vi "JME Test Solutions Visa Device Simulator.vi"() -> ()   [LabVIEW 2020]
doc: "This VI will wait for a TCP Connection and then respond to TCP Reqests based on the responses list"
panel:
  in  "Enable?":bool
  in  "Responses Config":string[][](array[string])
  in  "Load Button":bool
  in  "Responses File":path
  in  "stop":bool
  in  "port":u16=50000
  in  "Stop Button":bool
  # "JME Test Solutions VISA Device Simulator"
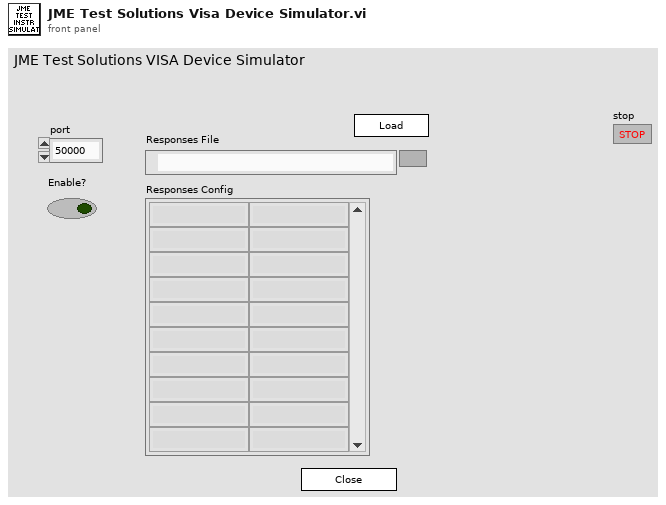
[diagram p1: front panel]
types:
  T1 = enum16{"Standard", "Buffered", "CRLF", "Immediate"}
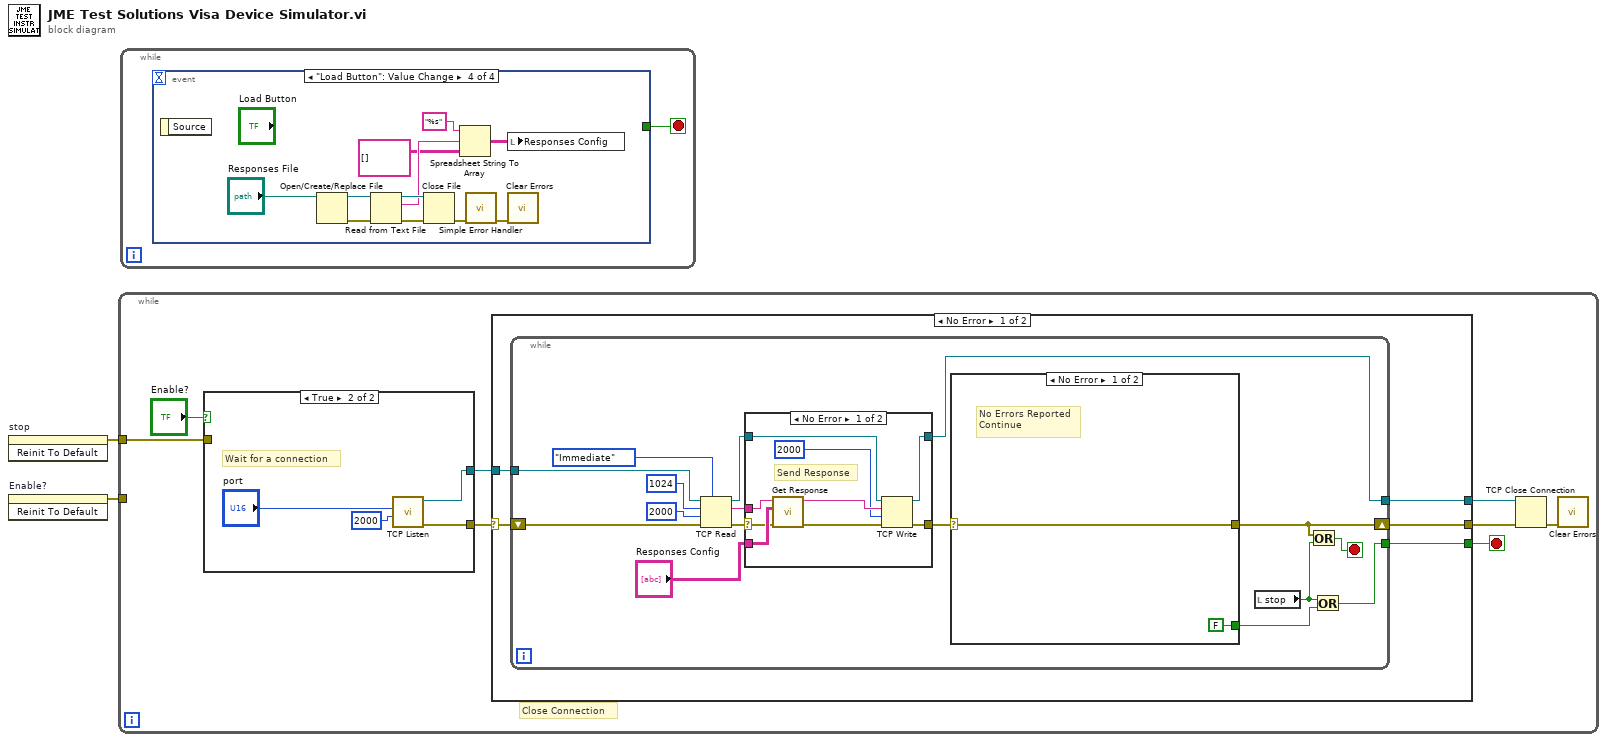
[diagram p0: block diagram]
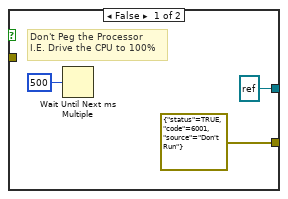
[diagram p2: hidden frame]
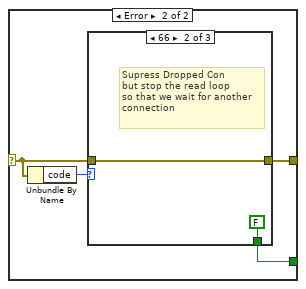
[diagram p3: hidden frame]
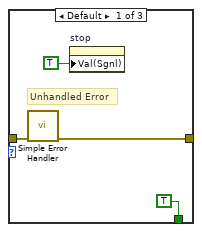
[diagram p4: hidden frame]
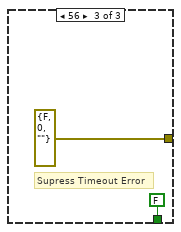
[diagram p5: hidden frame]
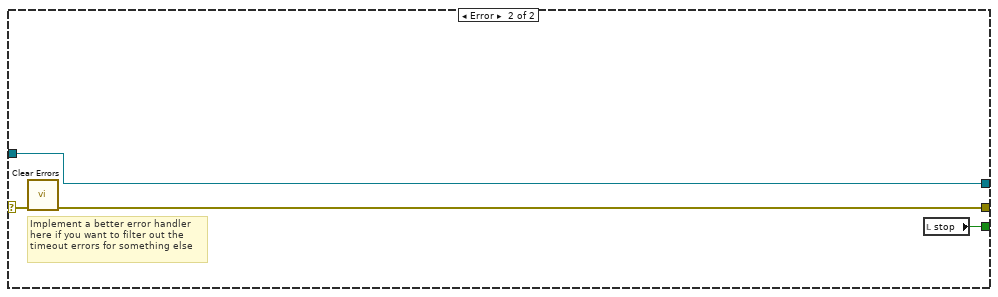
[diagram p7: hidden frame]
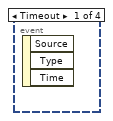
[diagram p8: hidden frame]
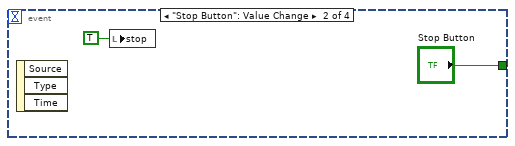
[diagram p9: hidden frame]
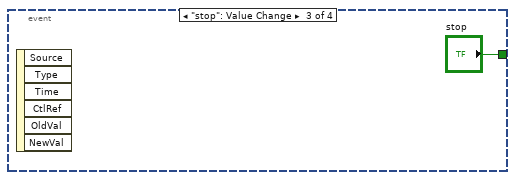
[diagram p10: hidden frame]
diagram:
  n1 = invoke on="stop" class="Bool (strict)" method="Reinit To Default"() -> (error out=w2:errorcluster)  [unwired: 3 in, 2 out]
  n2 = invoke on="Enable?" class="Bool (strict)" method="Reinit To Default"() -> (error out=w1:errorcluster)  [unwired: 3 in, 2 out]
  n3 = while {
    tunnel: w2 -> [w3]
    tunnel: w1 -> [_]
    stop <- w5 stop-if-true
    # "Close Connection"
    n4 = case shown="True" "Enable?" {
      tunnel: [errorcluster {"status"=TRUE, "code"=6001, "source"="Don't Run"} ("error out") w15] -> w10
      tunnel: [refnum<k5> refnum ("connection ID") w14] -> w9
      tunnel: w3 -> [_ _]
      frame False {
        # "Don't Peg the Processor\nI.E. Drive the CPU to 100%"
        n5 = Wait Until Next ms Multiple(millisecond multiple=u32 500) -> ()  [unwired: 1 out]
      }
      frame True {
        # "Wait for a connection"
        n6 = call <vilib>:"TCP Listen.vi"("timeout ms (wait forever: -1)"=2000, "port"="port") -> ("error out"=w15:errorcluster, "connection ID"=w14:refnum<k5>)  [unwired: 5 in, 3 out]
      }
    }
    n7 = case shown="No Error" w10 {
      selector: w10 -> [w21 w67]
      tunnel: w9 -> [w22 w66]
      tunnel: [w20 w66] -> w8
      tunnel: [w19 w65] -> w7
      tunnel: [w18 w64] -> w5
      frame No Error {
        n8 = while {
          tunnel: w22 -> [w38]
          shift-right: [w26] -> w19
          shift-left: w21 -> [w37]
          tunnel: [w28] -> w20
          tunnel: [w23] -> w18
          stop <- w30 stop-if-true
          n9 = TCP Read(connection ID=w38, bytes to read=1024, error in (no error)=w37, 7:T1."Immediate" ("mode (standard)"), 9:2000 ("timeout ms (25000)")) -> (connection ID out=w33:refnum<k5>, data out=w32:string, error out=w34:errorcluster)
          n10 = case shown="No Error" w34 {
            selector: w34 -> [w59 w62]
            tunnel: [w55 w62] -> w27
            tunnel: w33 -> [w57 w63]
            tunnel: [w56 w63] -> w28
            tunnel: w32 -> [w61 _]
            tunnel: "Responses Config" -> [w60 _]
            frame No Error {
              # "Send Response"
              n11 = call "Get Response.vi"("error in (no error)"=w59, "Responses Config"=w60, "Request"=w61) -> ("error out"=w58:errorcluster, "Response"=w54:string)  [unwired: 7 in]
              n12 = TCP Write(connection ID=w57, data in=w54, error in (no error)=w58, 9:2000 ("timeout ms (25000)")) -> (connection ID out=w56:refnum<k5>, error out=w55:errorcluster)  [unwired: 1 out]
            }
            frame Error {
            }
          }
          n13 = case shown="No Error" w27 {
            selector: w27 -> [w40 w43]
            tunnel: [w40 w42] -> w26
            tunnel: [FALSE ("x") w41] -> w24
            frame No Error {
              # "No Errors Reported\nContinue"
            }
            frame Error {
              n14 = Unbundle By Name(w43) -> ("code"=w44:i32)
              n15 = case shown="66" w44 {
                tunnel: w43 -> [w48 w50 _]
                tunnel: [w47 w50 errorcluster {"status"=FALSE, "code"=0, "source"=""} ("error IO")] -> w42
                tunnel: [TRUE ("x") FALSE ("x") FALSE ("x")] -> w41
                frame Default {
                  # "Unhandled Error"
                  n16 = call <vilib>:"Simple Error Handler.vi"("error in (no error)"=w48) -> ("error out"=w47:errorcluster)  [unwired: 4 in, 4 out]
                  n17 = property on="stop" class="Bool (strict)"("Val(Sgnl)"=TRUE ("Value (Signaling)")) -> ()  [unwired: 2 in, 2 out]
                }
                frame 66 {
                  # "Supress Dropped Con\nbut stop the read loop\nso that we wait for another\nconnection"
                }
                frame 56 {
                  # "Supress Timeout Error"
                }
              }
            }
          }
          n18 = local read "stop"() -> (w25:bool)
          n19 = Or(x=w26, y=w25) -> (x .or. y?=w30:bool)
          n20 = Or(x=w25, y=w24) -> (x .or. y?=w23:bool)
        }
      }
      frame Error {
        # "Implement a better error handler\nhere if you want to filter out the\ntimeout errors for something else"
        n21 = call <vilib>:"Clear Errors.vi"("error in (no error)"=w67) -> ("error out"=w65:errorcluster)  [unwired: 5 in, 1 out]
        n22 = local read "stop"() -> (w64:bool)
      }
    }
    n23 = TCP Close Connection(connection ID=w8, error in (no error)=w7) -> (error out=w6:errorcluster)  [unwired: 1 in, 1 out]
    n24 = call <vilib>:"Clear Errors.vi"("error in (no error)"=w6) -> ()  [unwired: 5 in, 2 out]
  }
  n25 = while {
    stop <- w68 stop-if-true
    n26 = event shown="[3] \"Load Button\": Value Change" {
      selector: _ -> [_ _ _ _]
      dyn-events: _ -> [_ _ _ _]
      timeout: _ -> [_ _ _ _]
      tunnel: [_ "Stop Button" "stop" _] -> w68
      event Timeout {
        n27 = event-data() -> ()  [unwired: 1 in, 3 out]
      }
      event "Stop Button": Value Change {
        n28 = event-data() -> ()  [unwired: 1 in, 3 out]
        n29 = local write "stop"(TRUE ("stop")) -> ()
      }
      event "stop": Value Change {
        n30 = event-data() -> ()  [unwired: 1 in, 6 out]
      }
      event "Load Button": Value Change {
        n31 = event-data() -> ()  [unwired: 1 in, 1 out]
        n32 = Open/Create/Replace File(file path (use dialog)="Responses File") -> (refnum out=w80:refnum<file>, error out=w81:errorcluster)  [unwired: 5 in, 1 out]
        n33 = Read from Text File(file (use dialog)=w80, error in=w81) -> (refnum out=w78:refnum<file>, text=w75:string, error out=w79:errorcluster)  [unwired: 2 in, 1 out]
        n34 = Close File(refnum=w78, error in=w79) -> (error out=w77:errorcluster)  [unwired: 1 out]
        n35 = Spreadsheet String To Array(format string="%s", spreadsheet string=w75, array type (2D Dbl)=string[][] []) -> (array=w72:string[][])  [unwired: 1 in]
        n36 = call <vilib>:"Simple Error Handler.vi"("error in (no error)"=w77) -> ("error out"=w76:errorcluster)  [unwired: 4 in, 4 out]
        n37 = local write "Responses Config"(w72) -> ()
        n38 = call <vilib>:"Clear Errors.vi"("error in (no error)"=w76) -> ()  [unwired: 5 in, 2 out]
      }
    }
  }
